vi "Variant to String.vi"(11 "Value":variant) -> (3 "String":string)   [LabVIEW 2020, in "Parallel Block.lvlib"]
uses:
  Parallel Block.lvlib
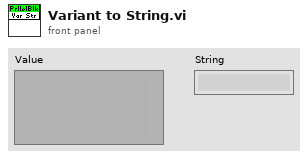
[diagram p1: front panel]
types:
  T1 = typedef "Parallel Block.lvlib/Value Type.ctl" = enum16{"Unknown", "Bool", "U8", "U16", "U32", "U64", "I8", "I16", "I32", "I64", "SGL", "DBL", "CSG", "CDB", "CDBWfm", "String", "DBLWfm"}
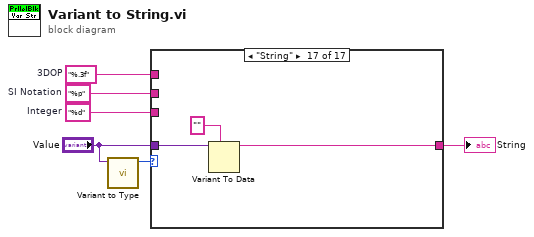
[diagram p0: block diagram]
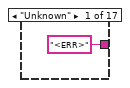
[diagram p2: hidden frame]
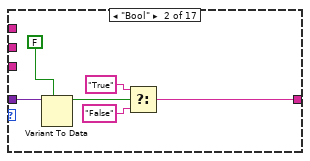
[diagram p3: hidden frame]
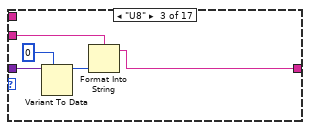
[diagram p4: hidden frame]
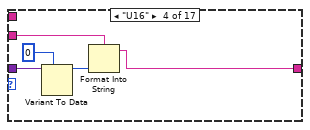
[diagram p5: hidden frame]
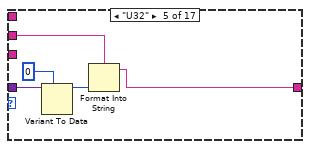
[diagram p6: hidden frame]
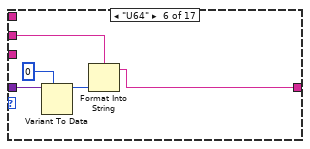
[diagram p7: hidden frame]
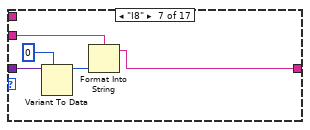
[diagram p8: hidden frame]
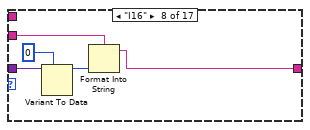
[diagram p9: hidden frame]
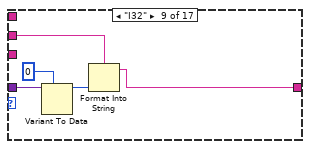
[diagram p10: hidden frame]
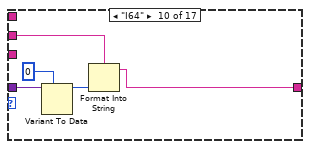
[diagram p11: hidden frame]
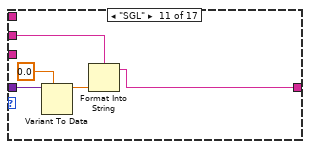
[diagram p12: hidden frame]
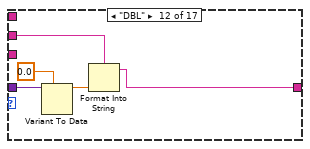
[diagram p13: hidden frame]
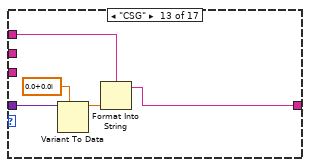
[diagram p14: hidden frame]
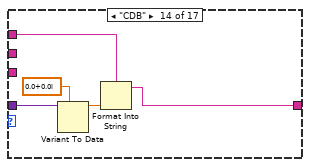
[diagram p15: hidden frame]
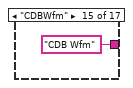
[diagram p16: hidden frame]
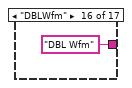
[diagram p17: hidden frame]
diagram:
  w1 = "%.3f"  # 3DOP
  w2 = "%p"  # SI Notation
  w3 = "%d"  # Integer
  n1 = call "Variant to Type.vi"("Value"="Value") -> ("Value Type"=w6:T1)  [unwired: 10 in]
  n2 = case shown="\"String\"" w6 {
    tunnel: "Value" -> [_ w13 w18 w23 w28 w33 w38 w43 w48 w53 w58 w63 w68 w73 _ _ w78]
    tunnel: ["<ERR>" w8 w14 w19 w24 w29 w34 w39 w45 w50 w55 w60 w65 w70 "CDB Wfm" "DBL Wfm" w76] -> w4
    tunnel: w3 -> [_ _ w15 w20 _ _ w35 w40 _ _ _ _ _ _ _ _ _]
    tunnel: w2 -> [_ _ _ _ w25 w30 _ _ w44 w49 w54 w59 _ _ _ _ _]
    tunnel: w1 -> [_ _ _ _ _ _ _ _ _ _ _ _ w64 w69 _ _ _]
    frame "Unknown" {
    }
    frame "Bool" {
      n3 = Variant To Data(type=FALSE, Variant=w13) -> (data=w11:bool)  [unwired: 1 in, 1 out]
      n4 = Select(t="True", s=w11, f="False") -> (s? t:f=w8:string)
    }
    frame "U8" {
      n5 = Variant To Data(type=u8 0, Variant=w18) -> (data=w16:u8)  [unwired: 1 in, 1 out]
      n6 = Format Into String(format string=w15, w16) -> (resulting string=w14:string)  [unwired: 2 in, 1 out]
    }
    frame "U16" {
      n7 = Variant To Data(type=u16 0, Variant=w23) -> (data=w21:u16)  [unwired: 1 in, 1 out]
      n8 = Format Into String(format string=w20, w21) -> (resulting string=w19:string)  [unwired: 2 in, 1 out]
    }
    frame "U32" {
      n9 = Variant To Data(type=u32 0, Variant=w28) -> (data=w26:u32)  [unwired: 1 in, 1 out]
      n10 = Format Into String(format string=w25, w26) -> (resulting string=w24:string)  [unwired: 2 in, 1 out]
    }
    frame "U64" {
      n11 = Variant To Data(type=u64 0, Variant=w33) -> (data=w31:u64)  [unwired: 1 in, 1 out]
      n12 = Format Into String(format string=w30, w31) -> (resulting string=w29:string)  [unwired: 2 in, 1 out]
    }
    frame "I8" {
      n13 = Variant To Data(type=i8 0, Variant=w38) -> (data=w36:i8)  [unwired: 1 in, 1 out]
      n14 = Format Into String(format string=w35, w36) -> (resulting string=w34:string)  [unwired: 2 in, 1 out]
    }
    frame "I16" {
      n15 = Variant To Data(type=i16 0, Variant=w43) -> (data=w41:i16)  [unwired: 1 in, 1 out]
      n16 = Format Into String(format string=w40, w41) -> (resulting string=w39:string)  [unwired: 2 in, 1 out]
    }
    frame "I32" {
      n17 = Variant To Data(type=0, Variant=w48) -> (data=w46:i32)  [unwired: 1 in, 1 out]
      n18 = Format Into String(format string=w44, w46) -> (resulting string=w45:string)  [unwired: 2 in, 1 out]
    }
    frame "I64" {
      n19 = Variant To Data(type=i64 0, Variant=w53) -> (data=w51:i64)  [unwired: 1 in, 1 out]
      n20 = Format Into String(format string=w49, w51) -> (resulting string=w50:string)  [unwired: 2 in, 1 out]
    }
    frame "SGL" {
      n21 = Variant To Data(type=sgl 0.0, Variant=w58) -> (data=w56:sgl)  [unwired: 1 in, 1 out]
      n22 = Format Into String(format string=w54, w56) -> (resulting string=w55:string)  [unwired: 2 in, 1 out]
    }
    frame "DBL" {
      n23 = Variant To Data(type=0.0, Variant=w63) -> (data=w61:dbl)  [unwired: 1 in, 1 out]
      n24 = Format Into String(format string=w59, w61) -> (resulting string=w60:string)  [unwired: 2 in, 1 out]
    }
    frame "CSG" {
      n25 = Variant To Data(type=csg 0.0+0.0i, Variant=w68) -> (data=w66:csg)  [unwired: 1 in, 1 out]
      n26 = Format Into String(format string=w64, w66) -> (resulting string=w65:string)  [unwired: 2 in, 1 out]
    }
    frame "CDB" {
      n27 = Variant To Data(type=cdb 0.0+0.0i, Variant=w73) -> (data=w71:cdb)  [unwired: 1 in, 1 out]
      n28 = Format Into String(format string=w69, w71) -> (resulting string=w70:string)  [unwired: 2 in, 1 out]
    }
    frame "CDBWfm" {
    }
    frame "DBLWfm" {
    }
    frame "String" {
      n29 = Variant To Data(type="", Variant=w78) -> (data=w76:string)  [unwired: 1 in, 1 out]
    }
  }
  "String" <- w4
